vi "Read Message Type.vi"(8 "error in (no error)":errorcluster, 11 "bt_WaitOn_Queue in":refnum<class "bt_WaitOn_Notifier.lvclass">) -> (0 "error out":errorcluster, 2 "Message Type":variant, 3 "bt_WaitOn_Queue out":refnum<class "bt_WaitOn_Notifier.lvclass">)   [LabVIEW 2021, in "BT.lvlib" / "bt_WaitOn_Notifier.lvclass"]
uses:
  bt_WaitOn_Notifier.lvclass
  bt_WaitOn_Notifier.lvclass/bt_WaitOn_Notifier.ctl
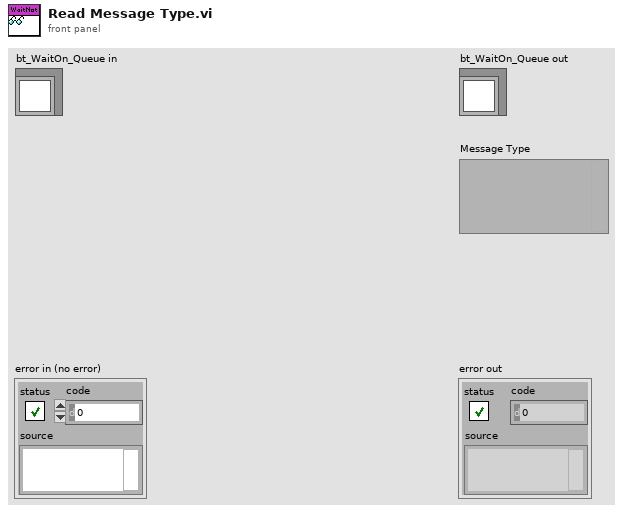
[diagram p1: front panel]
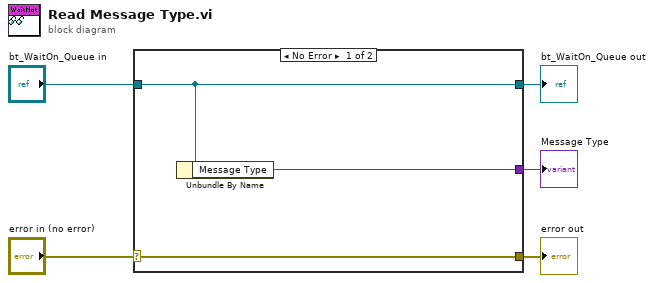
[diagram p0: block diagram]
diagram:
  n1 = case shown="No Error" "error in (no error)" {
    selector: "error in (no error)" -> [w8 w9]
    tunnel: [w8 w9] -> w4
    tunnel: [w7 w10] -> w2
    tunnel: "bt_WaitOn_Queue in" -> [w7 w10]
    tunnel: [w6 _] -> w1
    frame No Error {
      n2 = Unbundle By Name(w7) -> ("Message Type"=w6:variant)
    }
    frame Error {
    }
  }
  "error out" <- w4
  "bt_WaitOn_Queue out" <- w2
  "Message Type" <- w1
